vi "Measure.vi"(6 "error in (no error)":errorcluster, 9 "Generic Power Analyzer in":refnum<class "Generic Power Analyzer.lvclass">) -> (0 "error out":errorcluster, 2 "Array of Measurement":dbl[](array[numeric]), 3 "Generic Power Analyzer out":refnum<class "Generic Power Analyzer.lvclass">)   [LabVIEW 2014, in "Generic Power Analyzer.lvlib" / "Generic Power Analyzer.lvclass"]
uses:
  Generic Power Analyzer.lvclass
  Abstract Sensor/Abstract Sensor.lvclass
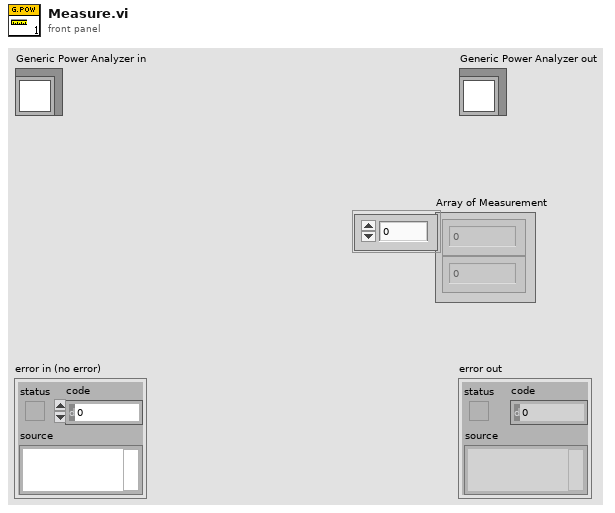
[diagram p1: front panel]
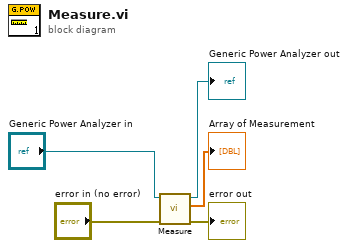
[diagram p0: block diagram]
diagram:
  n1 = call-parent "Measure.vi"("error in (no error)"="error in (no error)", "Abstract Sensor in"="Generic Power Analyzer in") -> ("error out"=→"error out":errorcluster, "Array of Measurement"=→"Array of Measurement":dbl[], "Abstract Sensor out"=→"Generic Power Analyzer out":refnum<class "Generic Power Analyzer.lvclass">)  [unwired: 5 in]
